vi "ZK断电保存全局变量.vi"() -> ()   [LabVIEW 2016, in "质控单元V4.lvlib"]
panel:
  in  "氟化物质控参数":T1={"量程"=100.0, "检出限"=5.0, "加标前水样浓度"=0.0, "加标后水样浓度"=0.0, "加标水杯定容体积"=0.0, "加标母液浓度"=0.0, "加标体积"=0.0, "加标回收率"=0.0}
  in  "显示详细日志":bool
  in  "CODcr质控参数":T1={"量程"=100.0, "检出限"=5.0, "加标前水样浓度"=0.0, "加标后水样浓度"=0.0, "加标水杯定容体积"=0.0, "加标母液浓度"=0.0, "加标体积"=0.0, "加标回收率"=0.0}
  in  "CODMn质控参数":T1={"量程"=10.0, "检出限"=0.3, "加标前水样浓度"=0.0, "加标后水样浓度"=0.0, "加标水杯定容体积"=0.0, "加标母液浓度"=0.0, "加标体积"=0.0, "加标回收率"=0.0}
  in  "总氮质控参数":T1={"量程"=12.0, "检出限"=0.25, "加标前水样浓度"=0.0, "加标后水样浓度"=0.0, "加标水杯定容体积"=0.0, "加标母液浓度"=0.0, "加标体积"=0.0, "加标回收率"=0.0}
  in  "总磷质控参数":T1={"量程"=1.2, "检出限"=0.025, "加标前水样浓度"=0.0, "加标后水样浓度"=0.0, "加标水杯定容体积"=0.0, "加标母液浓度"=0.0, "加标体积"=0.0, "加标回收率"=0.0}
  in  "氨氮质控参数":T1={"量程"=1.2, "检出限"=0.025, "加标前水样浓度"=0.0, "加标后水样浓度"=0.0, "加标水杯定容体积"=0.0, "加标母液浓度"=0.0, "加标体积"=0.0, "加标回收率"=0.0}
  in  "启用参数":T2={"氨氮"=TRUE, "总磷"=TRUE, "总氮"=TRUE, "CODMn"=TRUE, "CODCr"=FALSE, "氟化物"=FALSE}
  in  "Tab Control 2":enum32{"Comm Settings"}(tab)
  in  "Open":bool
  in  "Close":bool
  in  "Type":enum16{"Serial", "TCP"}(ring) caption="Connection Type"
  in  "Tab Control":enum32{"Page 1", "Page 2"}(tab)
  in  "Retries":i32=1
  in  "Timeout (ms)":u32=1000
  in  "Flow Control":u16(ring) items=["None", "XON/XOFF", "RTS/CTS", "XON/XOFF & RTS/CTS", "DTR/DSR", "XON/XOFF & DTR/DSR"]
  in  "Parity":u16(ring) items=["None", "Odd", "Even", "Mark", "Space"]
  in  "Stop Bits":u16(ring)=10 items=["1.0"=10, "1.5"=15, "2.0"=20]
  in  "Baud Rate (bps)":u32(ring)=115200 items=["9600"=9600, "19200"=19200, "38400"=38400, "57600"=57600, "115200"=115200, "460800"=460800, "921600"=921600]
  in  "Slave Address":u8=1
  in  "Mode":enum16{"RTU", "ASCII"}(ring)
  in  "COM Port":refnum<visa-resource-name>="COM8"
  in  "TCP_Port":u16=502 caption="Port"
  in  "IP Address":string="192.168.1.207"
  in  "TCP_Timeout":i32=1000 caption="Timeout (ms)"
  in  "TCP_Slave ID":u8=255 caption="Slave ID" format="%.0x"
  # "Communication Settngs"
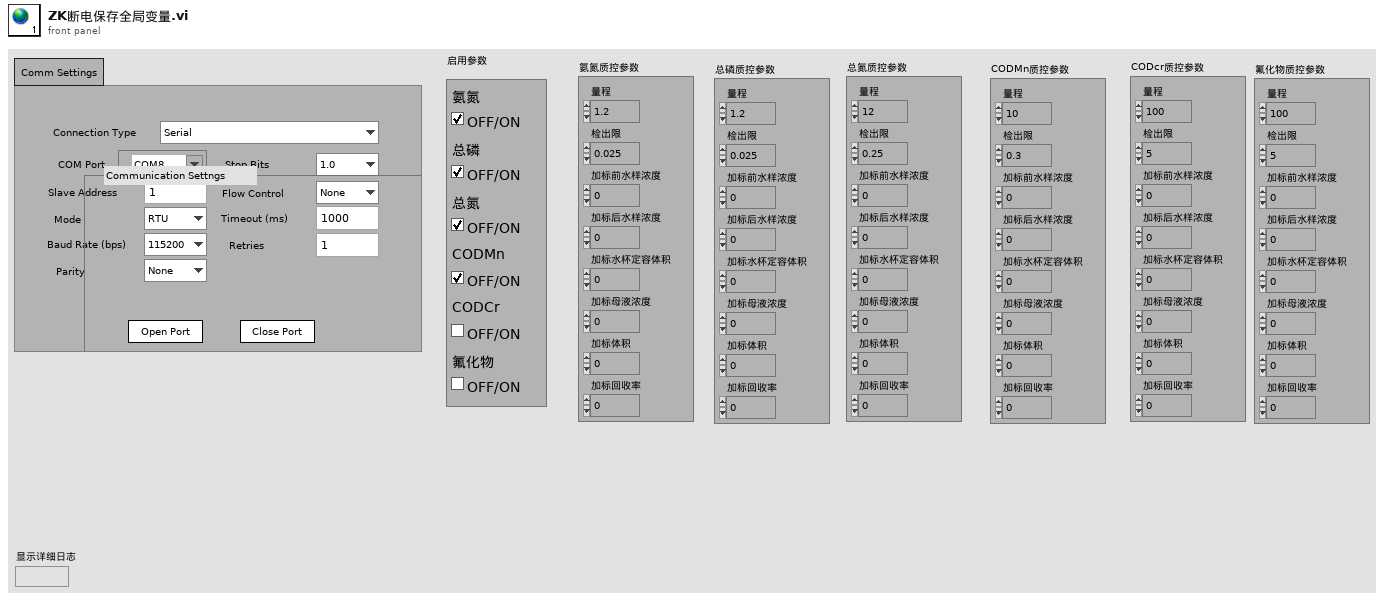
[diagram p1: front panel]
types:
  T1 = cluster{"量程":dbl, "检出限":dbl, "加标前水样浓度":dbl, "加标后水样浓度":dbl, "加标水杯定容体积":dbl, "加标母液浓度":dbl, "加标体积":dbl, "加标回收率":dbl}
  T2 = cluster{"氨氮":bool, "总磷":bool, "总氮":bool, "CODMn":bool, "CODCr":bool, "氟化物":bool}
diagram:
